vi "Robot Global Data.vi"() -> ()   [LabVIEW 2015]
doc: "This global VI can contain as many global variables as you need. Place a control on the panel, give it a good name. To read or write to it from a VI, drag the icon to the diagram of that VI. You can also drag from the project. Click on the node to change which global you access. You shouldn't have multiple locations writing to a global or it will cause a race-condition."
uses:
  <vilib>/Rock Robotics/WPI/Camera/WPI_CameraImageSize.ctl
  <vilib>/Rock Robotics/WPI/DriverStation/WPI_DriverStationRobotMode2.ctl
panel:
  out "Relevant Data":T1(array[cluster])
  out "Shooting":cluster{bool, bool, bool}
  out "More Detection":T2(array[cluster])
  out "ms to process":u32
  out "Detected Totes":T3(array[cluster]) {"Normalized Rect"."Numeric 5" format="%#_2g"; "Normalized Rect"."Numeric 3" format="%#_2g"; "Normalized Rect"."Numeric 2" format="%#_2g"; "Normalized Rect"."Numeric" format="%#_2g"}
  out "What to do":string
  in  "Robot Mode":T4
  in  "image size":T5=enum."320x240"
  in  "Enable Vision":bool
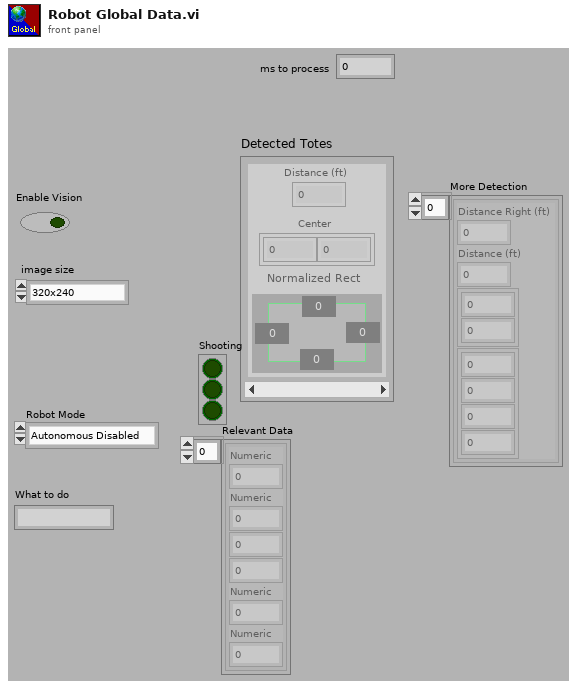
[diagram p1: front panel]
types:
  T1 = cluster{"Numeric":dbl, "Numeric":dbl, dbl, dbl, "Numeric":dbl, "Numeric":dbl}[]
  T2 = cluster{"Distance Right (ft)":dbl, "Distance (ft)":dbl, cluster{dbl, dbl}, cluster{dbl, dbl, dbl, dbl}}[]
  T3 = cluster{"Distance (ft)":dbl, "Center":cluster{dbl, dbl}, "Normalized Rect":cluster{"Numeric":dbl, "Numeric 2":dbl, "Numeric 3":dbl, "Numeric 5":dbl}}[]
  T4 = typedef "WPI_DriverStationRobotMode2.ctl" = enum16{"Autonomous Disabled", "Autonomous Enabled", "Teleop Disabled", "Teleop Enabled", "Disconnected", "Finish", "Test Disabled", "Test Enabled", "Emergency Stopped"}
  T5 = typedef "WPI_CameraImageSize.ctl" = enum16{"640x480", "320x240", "160x120", "Custom"}
diagram:
